vi "HRR-ajusteMatrix.vi"(8 "error in (no error)":errorcluster, 10 "Numero de motores":i32=8, 11 "file path (dialog if empty)":path) -> (0 "error out":errorcluster, 2 "output array":dbl[][][](array[numeric]), 3 "Matriz bruta":dbl[][](array[numeric]), 4 "numero de blocos":i32)   [LabVIEW 2019]
uses:
  <vilib>/Analysis/Matrix/Datatypes/RealMatrix.ctl
  <vilib>/Analysis/baseanly.llb/Real A x B.vi
  <vilib>/Utility/file.llb/Read Delimited Spreadsheet (DBL).vi
  <vilib>/Analysis/Matrix/Numeric/Conversions/Array To Matrix - RA2.vi
  <vilib>/Analysis/Matrix/Numeric/Conversions/Matrix To Array - RM.vi
  <vilib>/Analysis/Matrix/NI_Matrix.lvlib
  <vilib>/Analysis/NI_AALBase.lvlib
panel:
  in  "Inverte":dbl[][](array[numeric])=[[1.0, 1.0], [1.0, 1.0], [1.0, 1.0], [1.0, 1.0], [1.0, 1.0], [1.0, 1.0], [1.0, 1.0], [1.0, 1.0]]
  in  "Fator":T1=[[3.41, 0.0], [0.0, 8.973684210526317]] format="%#_11g"
  in  "Correção":dbl[][](array[numeric])=[[660.0, 0.0], [360.0, 0.0], [360.0, 0.0], [670.0, 0.0], [370.0, 0.0], [660.0, 0.0], [670.0, 0.0], [360.0, 0.0]]
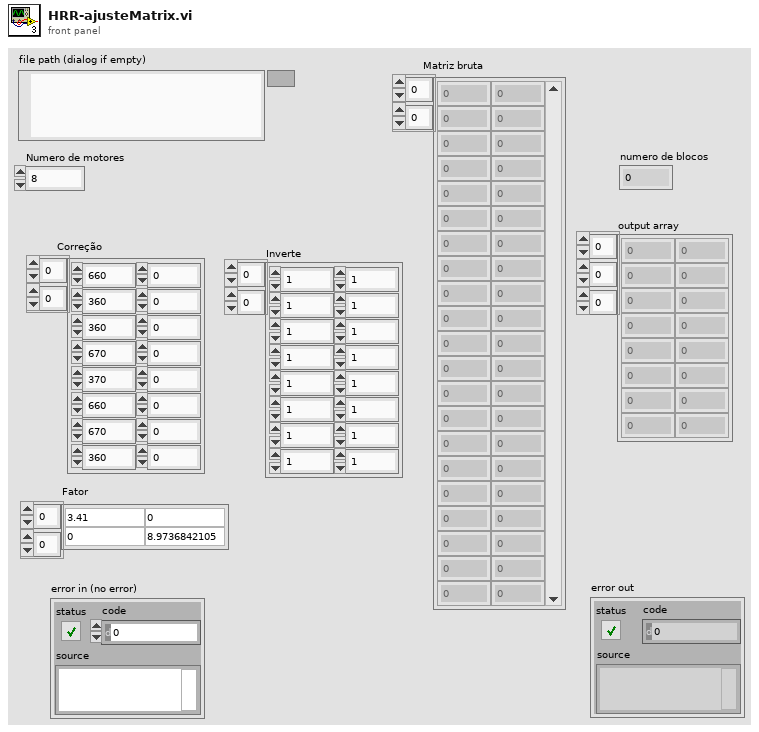
[diagram p1: front panel]
types:
  T1 = typedef "NI_Matrix.lvlib/RealMatrix.ctl" = dbl[][]
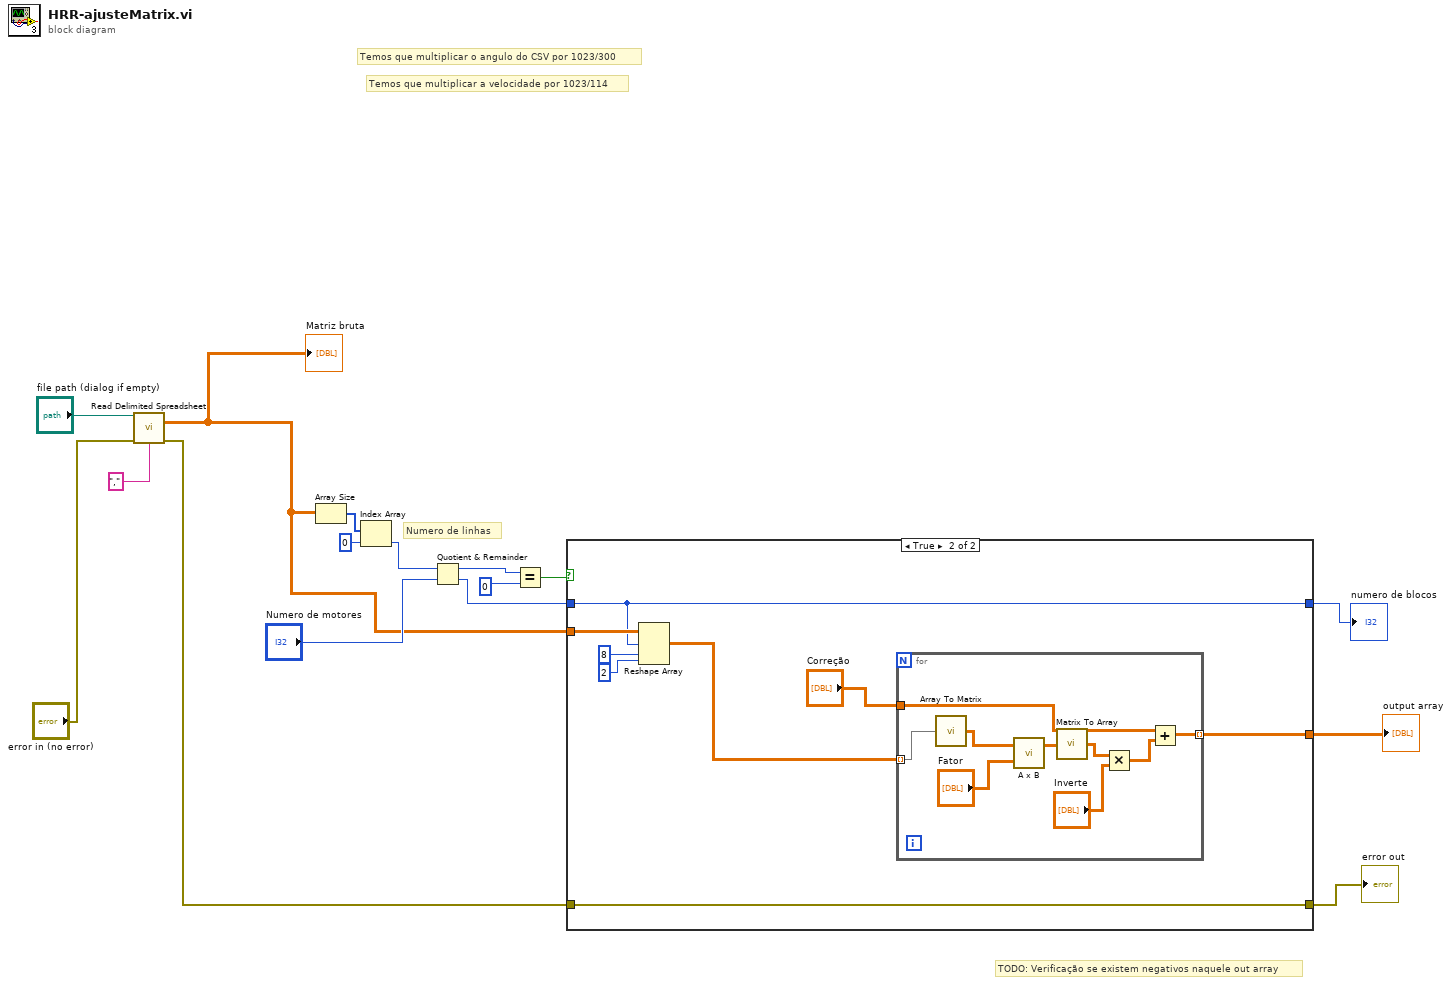
[diagram p0: block diagram]
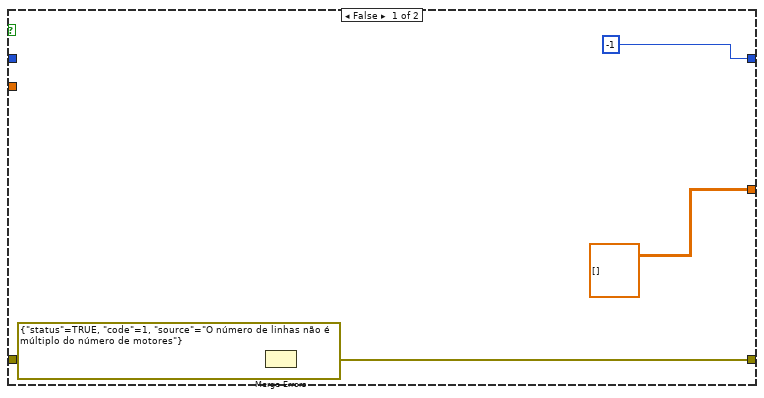
[diagram p2: hidden frame]
diagram:
  # "TODO: Verificação se existem negativos naquele out array"
  # "Temos que multiplicar a velocidade por 1023/114"
  # "Temos que multiplicar o angulo do CSV por 1023/300"
  # "Numero de linhas"
  n1 = call-poly <vilib>:"Read Delimited Spreadsheet.vi"("file path (dialog if empty)"="file path (dialog if empty)", "error in (no error)"="error in (no error)", "delimiter (\\t)"="," ("delimiter (\\t)")) -> ("all rows"=w3:dbl[][], "error out"=w5:errorcluster)  [unwired: 7 in, 4 out]
  "Matriz bruta" <- w3
  n2 = Array Size(array=w3) -> (size(s)=w15:i32[])
  n3 = Index Array(array=w15, index=0) -> (element=w14:i32)
  n4 = Quotient & Remainder(x=w14, y="Numero de motores") -> (x-y*floor(x/y)=w4:i32, floor(x/y)=w2:i32)
  n5 = Equal?(x=w4, y=0) -> (x = y?=w11:bool)
  n6 = case shown="True" w11 {
    tunnel: w2 -> [_ w24]
    tunnel: [-1 w24] -> w10
    tunnel: w5 -> [w20 w29]
    tunnel: [w19 w29] -> w9
    tunnel: w3 -> [_ w28]
    tunnel: [dbl[][][] [] w25] -> w1
    frame False {
      n7 = Merge Errors(errorcluster {"status"=TRUE, "code"=1, "source"="O número de linhas não é múltiplo do número de motores"} ("error in"), w20) -> (w19:errorcluster)
    }
    frame True {
      n8 = Reshape Array(w28, w24, 8 ("dimension size"), 2 ("dimension size")) -> (w26:dbl[][][])
      n9 = for {
        tunnel: w26 -> [w35] mode=indexing
        tunnel: "Correção" -> [w33]
        tunnel: [w34] -> w25 mode=indexing
        n10 = call-poly <vilib>:"Array To Matrix.vi"("Real 2D Array"=w35) -> ("Real Matrix"=w38:T1)
        n11 = call-poly <vilib>:"A x B.vi"("B"="Fator", "A"=w38) -> ("A x B"=w36:T1)  [unwired: 1 out]
        n12 = call-poly <vilib>:"Matrix To Array.vi"("Real Matrix"=w36) -> ("Real 2D Array"=w32:dbl[][])
        n13 = Multiply(x=w32, y="Inverte") -> (x*y=w31:dbl[][])
        n14 = Add(x=w33, y=w31) -> (x+y=w34:dbl[][])
      }
    }
  }
  "numero de blocos" <- w10
  "error out" <- w9
  "output array" <- w1
